vi "loadConfigFile.vi"(8 "error in":errorcluster, 10 "FilePathFast":T1) -> (0 "error out":errorcluster, 2 "ThetaLambdaMeanln10f":T2)   [LabVIEW 2016]
uses:
  <vilib>/Utility/config.llb/Read Key (Double).vi
  <vilib>/Utility/config.llb/NI_LVConfig.lvlib
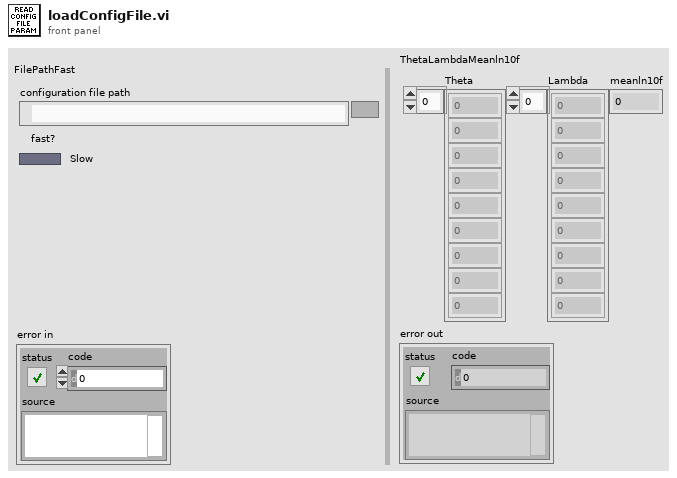
[diagram p1: front panel]
types:
  T1 = cluster{"configuration file path":path, "fast?":bool}
  T2 = cluster{"Theta":dbl[], "Lambda":dbl[], "meanln10f":dbl}
  T3 = typedef "NI_LVConfig.lvlib/Config Data RefNum.ctl" = refnum<k1>
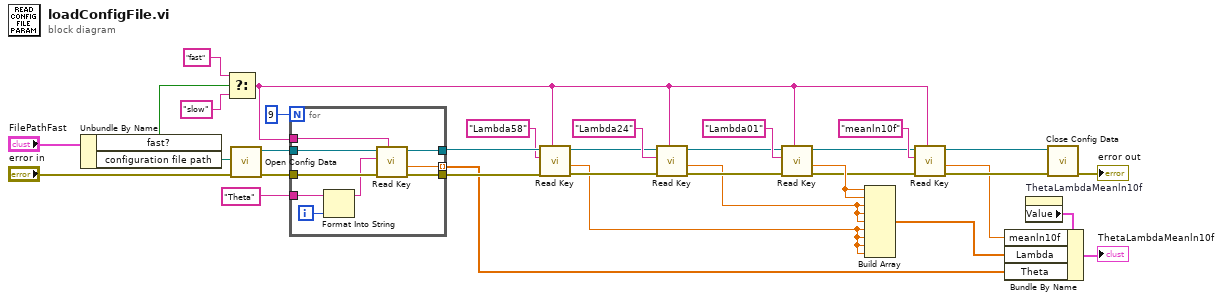
[diagram p0: block diagram]
diagram:
  n1 = Unbundle By Name("FilePathFast") -> ("fast?"=w4:bool, "configuration file path"=w5:path)
  n2 = Select(t="fast", s=w4, f="slow") -> (s? t:f=w14:string)
  n3 = call <vilib>:"Open Config Data.vi"("error in (no error)"="error in", "configuration file path"=w5) -> ("error out"=w32:errorcluster, "refnum"=w34:T3)  [unwired: 7 in, 1 out]
  n4 = for {
    N: 9 -> [_]
    tunnel: w34 -> [w43]
    tunnel: [w42] -> w28
    tunnel: [w41] -> w7 mode=indexing
    tunnel: w32 -> [w40]
    tunnel: [w39] -> w29
    tunnel: w14 -> [w38]
    tunnel: "Theta" ("initial string") -> [w35]
    i -> [w37]
    n5 = Format Into String(initial string=w35, w37) -> (resulting string=w36:string)  [unwired: 2 in, 1 out]
    n6 = call-poly <vilib>:"Read Key.vi"("section"=w38, "error in (no error)"=w40, "key"=w36, "refnum"=w43) -> ("error out"=w39:errorcluster, "value"=w41:dbl, "refnum out"=w42:T3)  [unwired: 4 in, 1 out]
  }
  n7 = call-poly <vilib>:"Read Key.vi"("section"=w14, "error in (no error)"=w29, "key"="Lambda58", "refnum"=w28) -> ("error out"=w23:errorcluster, "value"=w18:dbl, "refnum out"=w24:T3)  [unwired: 4 in, 1 out]
  n8 = call-poly <vilib>:"Read Key.vi"("section"=w14, "error in (no error)"=w23, "key"="Lambda24", "refnum"=w24) -> ("error out"=w22:errorcluster, "value"=w19:dbl, "refnum out"=w21:T3)  [unwired: 4 in, 1 out]
  n9 = call-poly <vilib>:"Read Key.vi"("section"=w14, "error in (no error)"=w22, "key"="Lambda01", "refnum"=w21) -> ("error out"=w16:errorcluster, "value"=w20:dbl, "refnum out"=w15:T3)  [unwired: 4 in, 1 out]
  n10 = Build Array(w20, w20, w19, w19, w19, w18, w18, w18, w18) -> (w8:dbl[])
  n11 = call-poly <vilib>:"Read Key.vi"("section"=w14, "error in (no error)"=w16, "key"="meanln10f", "refnum"=w15) -> ("error out"=w13:errorcluster, "value"=w9:dbl, "refnum out"=w12:T3)  [unwired: 4 in, 1 out]
  n12 = property on="ThetaLambdaMeanln10f" class="Clust (strict)"() -> ("Value"=w10:T2)  [unwired: 2 in, 2 out]
  n13 = Bundle By Name(cluster=w10, "meanln10f"=w9, "Lambda"=w8, "Theta"=w7) -> (→"ThetaLambdaMeanln10f":T2)
  n14 = call <vilib>:"Close Config Data.vi"("error in (no error)"=w13, "refnum"=w12) -> ("error out"=→"error out":errorcluster)  [unwired: 8 in, 1 out]
